vi "Check String Type.vi"(8 "error in (no error)":errorcluster, 10 "String":string, 11 "Numeric Value in":refnum<class "Numeric Value.lvclass">) -> (0 "error out":errorcluster, 3 "Numeric Value out":refnum<class "Numeric Value.lvclass">)   [LabVIEW 2020, in "Composed Columns.lvlib" / "Numeric Value.lvclass"]
uses:
  Numeric Value.lvclass
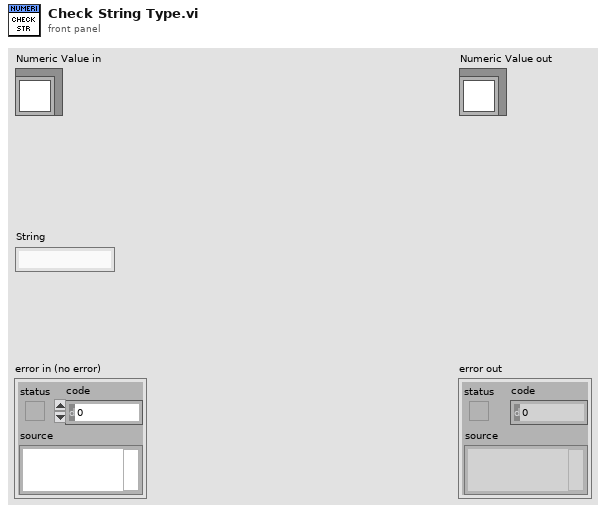
[diagram p1: front panel]
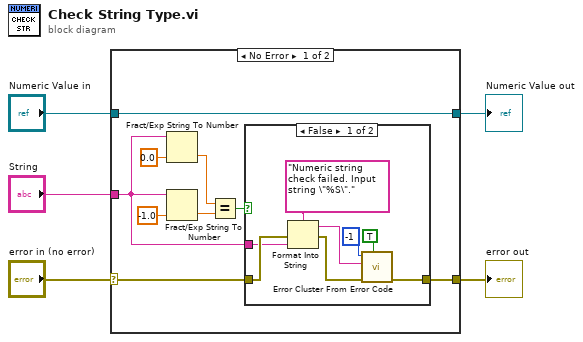
[diagram p0: block diagram]
diagram:
  n1 = case shown="No Error" "error in (no error)" {
    selector: "error in (no error)" -> [w9 w25]
    tunnel: [w8 w25] -> w4
    tunnel: "Numeric Value in" -> [w7 w24]
    tunnel: [w7 w24] -> w2
    tunnel: "String" -> [w6 _]
    frame No Error {
      n2 = Fract/Exp String To Number(string=w6, default (0 dbl)=0.0 ("default (0 DBL)")) -> (number=w11:dbl)  [unwired: 2 in, 1 out]
      n3 = Fract/Exp String To Number(string=w6, default (0 dbl)=-1.0 ("default (0 DBL)")) -> (number=w12:dbl)  [unwired: 2 in, 1 out]
      n4 = Equal?(x=w11, y=w12) -> (x = y?=w10:bool)
      n5 = case shown="False" w10 {
        tunnel: w9 -> [w21 w23]
        tunnel: [w19 w23] -> w8
        tunnel: w6 -> [w15 _]
        frame False {
          n6 = Format Into String(format string="Numeric string check failed. Input string \"%S\".", error in=w21, w15) -> (resulting string=w18:string, error out=w20:errorcluster)  [unwired: 1 in]
          n7 = call <vilib>:"Error Cluster From Error Code.vi"("show call chain? (False)"=TRUE, "error in (no error)"=w20, "error message (\"\")"=w18, "error code (0)"=-1) -> ("error out"=w19:errorcluster)  [unwired: 5 in]
        }
        frame True {
        }
      }
    }
    frame Error {
    }
  }
  "error out" <- w4
  "Numeric Value out" <- w2
